vi "Read INI File.vi"(8 "error in (no error)":errorcluster, 10 "section":string, 11 "ini file path":path) -> (0 "error out":errorcluster, 2 "keyed array":T1, 3 "duplicate ini file path":path)   [LabVIEW 2020, in "NI_FTP.lvlib"]
uses:
  <vilib>/FTP/NI_FTP.lvlib
  <vilib>/FTP/util/Keyed Array.ctl
panel:
  in  "empty keyed array":T1
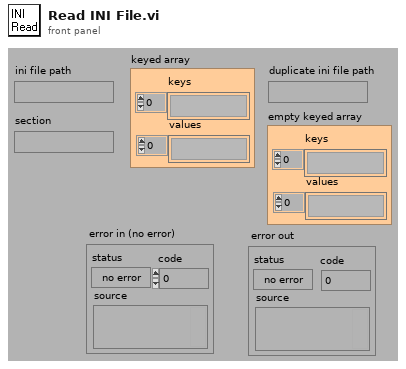
[diagram p1: front panel]
types:
  T1 = typedef "NI_FTP.lvlib/Keyed Array.ctl" = cluster{"keys":string[], "values":string[]}
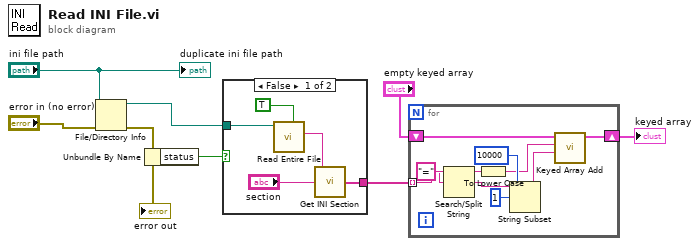
[diagram p0: block diagram]
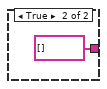
[diagram p2: hidden frame]
diagram:
  n1 = File/Directory Info(path="ini file path", error in="error in (no error)") -> (path out=w3:path, error out=w5:errorcluster)  [unwired: 5 out]
  "error out" <- w5
  n2 = Unbundle By Name(w5) -> ("status"=w4:bool)
  n3 = case shown="False" w4 {
    tunnel: w3 -> [w13 _]
    tunnel: [w12 string[] [] ("section")] -> w8
    frame False {
      n4 = call <vilib>:"Read Entire File.vi"("convert eoln (F)"=TRUE ("convert eol? (no:F)"), "path"=w13) -> ("data"=w9:string)  [unwired: 1 in, 8 out]
      n5 = call <vilib>:"Get INI Section.vi"("section name"="section", "file content"=w9) -> ("section"=w12:string[])  [unwired: 3 out]
    }
    frame True {
    }
  }
  n6 = for {
    tunnel: w8 -> [w24] mode=indexing
    shift-right: [w16] -> w6
    shift-left: "empty keyed array" -> [w18]
    n7 = Search/Split String(string=w24, search string/char (-)="=" ("search char (-)")) -> (substring before match=w22:string, match + rest of string=w21:string)  [unwired: 2 out]
    n8 = To Lower Case(string=w22) -> (all lower case string=w15:string)
    n9 = String Subset(string=w21, offset (0)=1, length (rest)=10000 ("offset (0)")) -> (substring=w17:string)
    n10 = call <vilib>:"Keyed Array Add.vi"("value"=w17, "key"=w15, "array in"=w18) -> ("array out"=w16:T1)  [unwired: 1 in, 3 out]
  }
  "keyed array" <- w6
  "duplicate ini file path" <- "ini file path"
